vi "Save Accel Data.vi"(8 "error in (no error)":errorcluster, 11 "Accel Config":T1={"PS Sens"=0.0001, "GB Sens"=0.0001, "FAN Sens"=0.0001, "PS Cutoff Frequency"={"LP Passband"=1200.0, "HP Stopband"=250.0, "LP Stopband"=1300.0, "HP Passband"=300.0}, "GB Cutoff Frequency"={"LP Passband"=1200.0, "HP Stopband"=250.0, "LP Stopband"=1300.0, "HP Passband"=300.0}, "Fan Cutoff Frequency"={"LP Passband"=1200.0, "HP Stopband"=250.0, "LP Stopband"=1300.0, "HP Passband"=300.0}} {"PS Cutoff Frequency"."HP Passband" min=1.0 step=1.0 format="%#.4f"; "PS Cutoff Frequency"."LP Stopband" min=1.0 step=1.0 format="%#.4f"; "PS Cutoff Frequency"."HP Stopband" min=1.0 step=1.0 format="%#.4f"; "PS Cutoff Frequency"."LP Passband" min=1.0 step=1.0 format="%#.4f"; "GB Cutoff Frequency"."HP Passband" min=1.0 step=1.0 format="%#.4f"; "GB Cutoff Frequency"."LP Stopband" min=1.0 step=1.0 format="%#.4f"; "GB Cutoff Frequency"."HP Stopband" min=1.0 step=1.0 format="%#.4f"; "GB Cutoff Frequency"."LP Passband" min=1.0 step=1.0 format="%#.4f"; "Fan Cutoff Frequency"."HP Passband" min=1.0 step=1.0 format="%#.4f"; "Fan Cutoff Frequency"."LP Stopband" min=1.0 step=1.0 format="%#.4f"; "Fan Cutoff Frequency"."HP Stopband" min=1.0 step=1.0 format="%#.4f"; "Fan Cutoff Frequency"."LP Passband" min=1.0 step=1.0 format="%#.4f"}) -> (0 "error out":errorcluster)   [LabVIEW 2018, in "File IO.lvlib"]
doc: "This subVI enqueues the named action in to the communications queue along with the input data."
uses:
  File IO.lvlib
  Testing UI 3/Public Controls/Accel Config.ctl
  Testing UI 3/Private Controls/Cutoff Frequency.ctl
  Private Controls/Module Data.ctl
  Private Controls/Module Action.ctl
  Testing UI 3/Testing UI 3.lvlib
panel:
  # "Highpass Cutoff Frequency"
  # "Lowpass Cutoff Frequency"
  # "Highpass Cutoff Frequency"
  # "Lowpass Cutoff Frequency"
  # "Highpass Cutoff Frequency"
  # "Lowpass Cutoff Frequency"
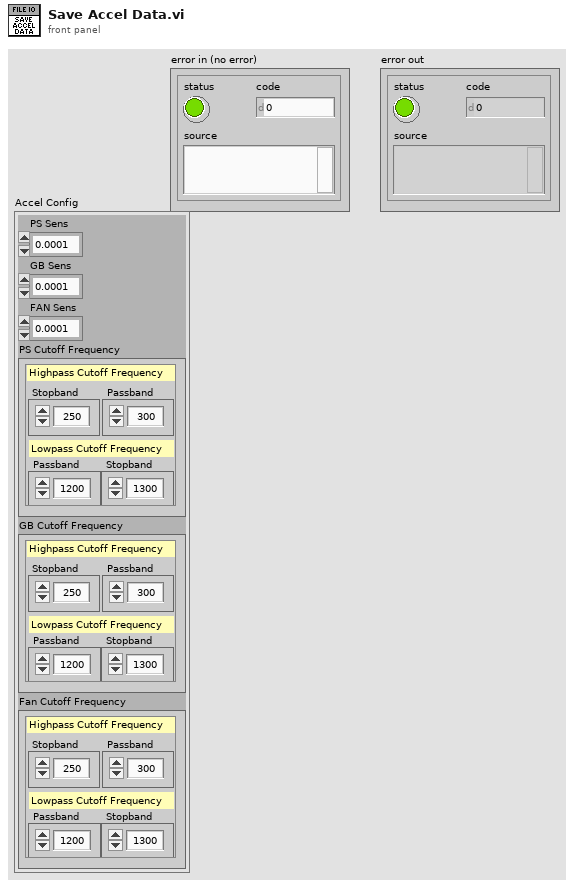
[diagram p1: front panel]
types:
  T1 = typedef "Testing UI 3.lvlib/Accel Config.ctl" = cluster{"PS Sens":dbl, "GB Sens":dbl, "FAN Sens":dbl, "PS Cutoff Frequency":T2, "GB Cutoff Frequency":T2, "Fan Cutoff Frequency":T2}
  T2 = typedef "Testing UI 3.lvlib/Cutoff Frequency.ctl" = cluster{"LP Passband":dbl, "HP Stopband":dbl, "LP Stopband":dbl, "HP Passband":dbl}
  T3 = typedef "File IO.lvlib/Module Action.ctl" = enum8{"Timeout", "OpenReport", "Continue Test", "Init", "Error", "Exit", "Save Accel Data", "Set Recording State", "Log APU RunTime", "Start New Test", "Create New Reports", "Write to System Log", "Save Variables", "Load APU Setup File", "Increment Run Count", "Write To Report"}
  T4 = typedef "File IO.lvlib/Module Data.ctl" = cluster{"Data":variant, "Action":T3}
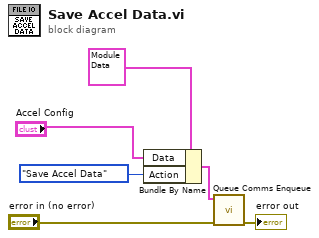
[diagram p0: block diagram]
diagram:
  n1 = Bundle By Name(cluster=T4 {"Data"=variant, "Action"=enum."Init"} ("element"), "Data"="Accel Config", "Action"=Module_Action."Save Accel Data") -> (w6:T4)
  n2 = call "Queue Comms Enqueue.vi"("error in (no error)"="error in (no error)", "element"=w6) -> ("error out"=→"error out":errorcluster)  [unwired: 9 in]
